vi "Scale to Absolute Pressure.vi"(9 "Pressure (psi atm)":dbl, 10 "Atm Press":dbl) -> (1 "Pressure out (psi atm)":dbl, 2 "Pressure (psi abs)":dbl)   [LabVIEW 2013]
doc: "This sub-VI scales atmospheric psi to absolute psi (fix this description)"
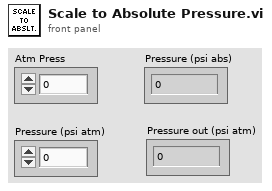
[diagram p1: front panel]
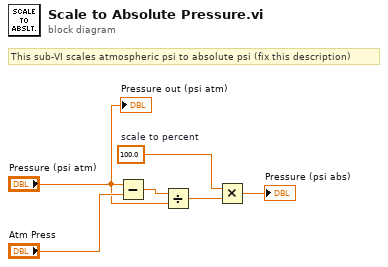
[diagram p0: block diagram]
diagram:
  w5 = 100.0  # scale to percent
  # "This sub-VI scales atmospheric psi to absolute psi (fix this description)"
  n1 = Subtract(x="Pressure (psi atm)", y="Atm Press") -> (x-y=w3:dbl)
  n2 = Divide(x=w3, y="Pressure (psi atm)") -> (x/y=w4:dbl)
  n3 = Multiply(x=w5, y=w4) -> (x*y=→"Pressure (psi abs)":dbl)
  "Pressure out (psi atm)" <- "Pressure (psi atm)"
